vi "Reset.vi"(8 "error in (no error)":errorcluster, 10 "Message in":refnum<class "ResetMessage.lvclass">, 11 "Waveform in":refnum<class "Waveform.lvclass">) -> (0 "error out":errorcluster, 3 "Waveform out":refnum<class "Waveform.lvclass">)   [LabVIEW 2012, in "Waveform.lvclass"]
doc: "The reset method processes the command 'reset'. \n\nResets the internal state of the component (without performing a full initialisation). This could be resetting hardware, or private data to default values."
uses:
  Waveform.lvclass
  <vilib>/Distrio/Murmex/Murmex/Murmex.lvclass
  <vilib>/Distrio/Murmex/StopMessage/StopMessage.lvclass
  <vilib>/Distrio/Murmex/StartMessage/StartMessage.lvclass
  <vilib>/Distrio/Murmex/ResetMessage/ResetMessage.lvclass
panel:
  # "This method is called when the RESET\ntrigger is sent. \n\nOverride this method when your component needs to\nrespond to this trigger. \n\nCall parent for proper implementation"
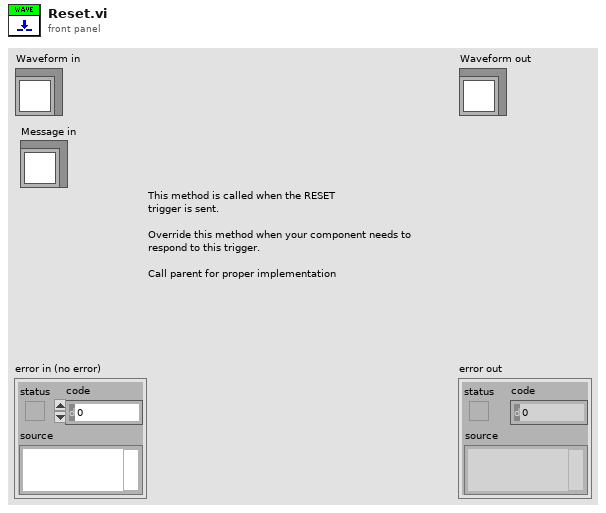
[diagram p1: front panel]
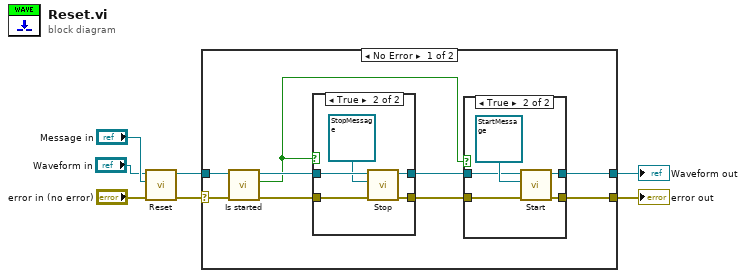
[diagram p0: block diagram]
diagram:
  n1 = call-parent "Reset.vi"("error in (no error)"="error in (no error)", "Message in"="Message in", "Murmex in"="Waveform in") -> ("error out"=w4:errorcluster, "Murmex out"=w2:refnum<class "Waveform.lvclass">)  [unwired: 7 in]
  n2 = case shown="No Error" w4 {
    selector: w4 -> [w16 w31]
    tunnel: [w9 w32] -> w3
    tunnel: w2 -> [w12 w32]
    tunnel: [w13 w31] -> w1
    frame No Error {
      n3 = call <vilib>:"Is started.vi"("error in (no error)"=w16, "Murmex in"=w12) -> ("error out"=w15:errorcluster, "started?"=w8:bool, "Murmex out"=w11:refnum<class "Waveform.lvclass">)  [unwired: 7 in]
      n4 = case shown="True" w8 {
        tunnel: w15 -> [w25 w30]
        tunnel: [w25 w29] -> w14
        tunnel: w11 -> [w24 w28]
        tunnel: [w24 w27] -> w10
        frame False {
        }
        frame True {
          n5 = call-dynamic "Stop.vi"("error in (no error)"=w30, "Message in"=refnum<class "StopMessage.lvclass"> refnum ("Murmex.lvlib:StopMessage"), "Waveform in"=w28) -> ("error out"=w29:errorcluster, "Waveform out"=w27:refnum<class "Waveform.lvclass">)  [unwired: 7 in]
        }
      }
      n6 = case shown="True" w8 {
        tunnel: w14 -> [w18 w19]
        tunnel: [w18 w22] -> w13
        tunnel: w10 -> [w17 w20]
        tunnel: [w17 w23] -> w9
        frame False {
        }
        frame True {
          n7 = call-dynamic "Start.vi"("error in (no error)"=w19, "Message in"=refnum<class "StartMessage.lvclass"> refnum ("Murmex.lvlib:StartMessage"), "Waveform in"=w20) -> ("error out"=w22:errorcluster, "Waveform out"=w23:refnum<class "Waveform.lvclass">)  [unwired: 7 in]
        }
      }
    }
    frame Error {
    }
  }
  "error out" <- w1
  "Waveform out" <- w3
